vi "Perform Action.vi"(8 "error in (no error)":errorcluster, 10 "Input":variant, 11 "Virtual Instrument in":refnum<class "Virt Voltage Reader.lvclass">) -> (0 "error out":errorcluster, 2 "Output":variant, 3 "Virtual Instrument out":refnum<class "Virt Voltage Reader.lvclass">)   [LabVIEW 2023, in "Virt Scopes.lvlib" / "Virt Voltage Reader.lvclass"]
uses:
  Virt Voltage Reader.lvclass
  Virt Voltage Reader.lvclass/Virt Voltage Reader.ctl
  <vilib>/Analysis/NI_AALBase.lvlib
  <vilib>/Analysis/baseanly.llb/Mean (DBL).vi
  Virt Instrument Base/Virt Instr Base.lvclass
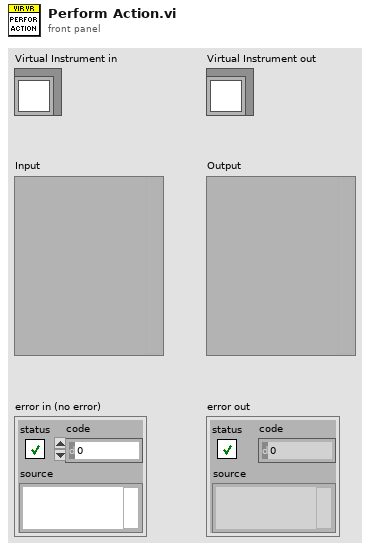
[diagram p1: front panel]
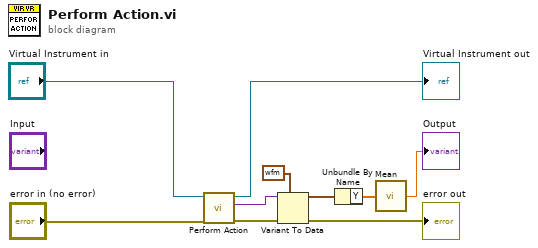
[diagram p0: block diagram]
diagram:
  n1 = call-parent "Perform Action.vi"("error in (no error)"="error in (no error)", "Virt Instrument Base in"="Virtual Instrument in") -> ("error out"=w8:errorcluster, "Output"=w6:variant, "Virt Instrument Base out"=→"Virtual Instrument out":refnum<class "Virt Voltage Reader.lvclass">)  [unwired: 7 in]
  n2 = Variant To Data(error in=w8, type=waveform(dbl) {"t0"=timestamp(0 s since 1904-01-01), "dt"=1.0, "Y"=[]} ("Waveform"), Variant=w6) -> (data=w5:waveform(dbl), error out=→"error out":errorcluster)
  n3 = Unbundle By Name(w5) -> ("Y"=w3:dbl[])
  n4 = call-poly <vilib>:"Mean.vi"("X"=w3) -> ("mean"=→"Output":dbl)  [unwired: 1 out]
